vi "PIDF.vi"() -> ()   [LabVIEW 2016]
panel:
  in  "i Zone":dbl format="%.2f"
  in  "Feed Forward":dbl format="%.2f"
  out "output":dbl format="%.2f"
  in  "setpoint":dbl format="%.2f"
  in  "process variable":dbl format="%.2f"
  in  "PIDF gains":cluster{"Kp":dbl, "Ki":dbl, "Kd":dbl, "Kf":dbl}={"Kp"=1.0, "Ki"=0.01, "Kd"=0.0, "Kf"=1.0} {"Kf" format="%.3f"; "Kd" format="%.3f"; "Ki" format="%.3f"; "Kp" format="%.3f"}
  in  "dt (s)":dbl=-1.0 format="%.3f"
  in  "output range":cluster{"output high":dbl, "output low":dbl}={"output high"=1.0, "output low"=-1.0} {"output low" format="%.2f"; "output high" format="%.2f"}
  in  "reinitialize? (F)":bool
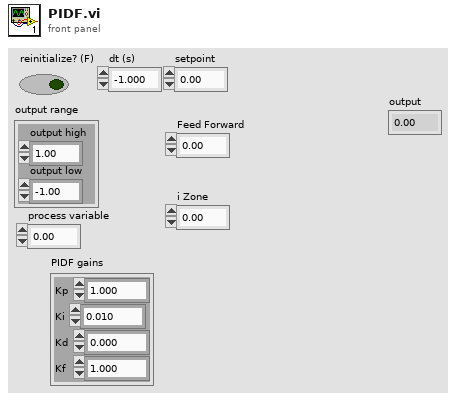
[diagram p1: front panel]
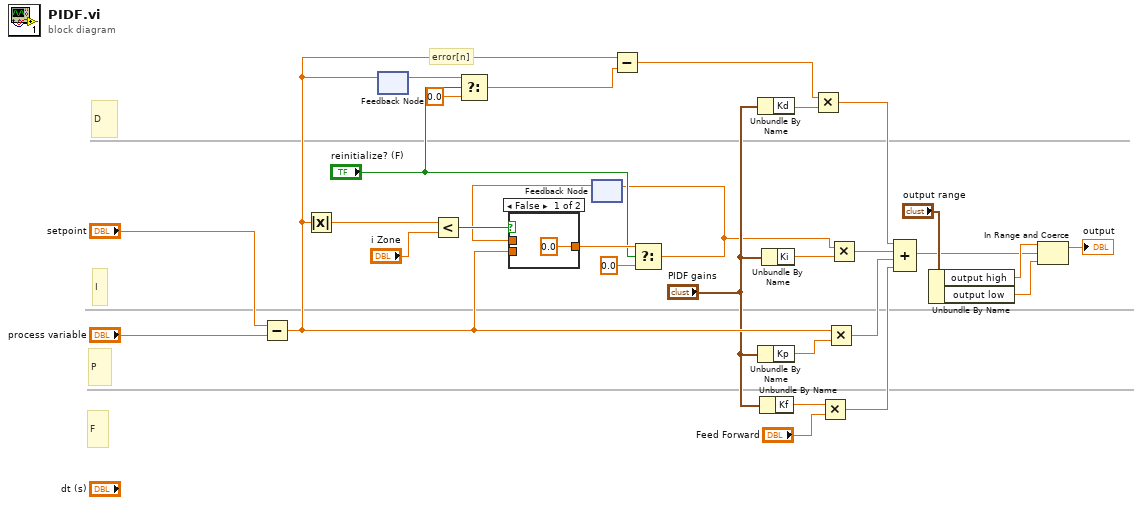
[diagram p0: block diagram]
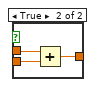
[diagram p2: hidden frame]
diagram:
  # "F"
  # "D"
  # "I"
  # "P"
  # "error[n]"
  n1 = Subtract(x="setpoint", y="process variable") -> (x-y=w20:dbl)
  n2 = Absolute Value(x=w20) -> (abs(x)=w27:dbl)
  n3 = feedback #1() -> (w18:dbl)  [unwired: 1 in]
  n4 = feedback-in #1(w20) -> ()
  n5 = Less?(x=w27, y="i Zone") -> (x < y?=w25:bool)
  n6 = Select(t=w18, s="reinitialize? (F)", f=0.0) -> (s? t:f=w17:dbl)
  n7 = feedback #2() -> (w24:dbl)  [unwired: 1 in]
  n8 = case shown="False" w25 {
    tunnel: w20 -> [_ w34]
    tunnel: [0.0 ("f") w33] -> w23
    tunnel: w24 -> [_ w32]
    frame False {
    }
    frame True {
      n9 = Add(x=w32, y=w34) -> (x+y=w33:dbl)
    }
  }
  n10 = Subtract(x=w20, y=w17) -> (x-y=w5:dbl)
  n11 = Select(t=w23, s="reinitialize? (F)", f=0.0) -> (s? t:f=w2:dbl)
  n12 = feedback-in #2(w2) -> ()
  n13 = Unbundle By Name("PIDF gains") -> ("Kd"=w6:dbl)
  n14 = Unbundle By Name("PIDF gains") -> ("Kp"=w28:dbl)
  n15 = Unbundle By Name("PIDF gains") -> ("Kf"=w9:dbl)
  n16 = Unbundle By Name("PIDF gains") -> ("Ki"=w3:dbl)
  n17 = Multiply(x=w5, y=w6) -> (x*y=w4:dbl)
  n18 = Multiply(x=w9, y="Feed Forward") -> (x*y=w7:dbl)
  n19 = Multiply(x=w20, y=w28) -> (x*y=w16:dbl)
  n20 = Multiply(x=w2, y=w3) -> (x*y=w1:dbl)
  n21 = Compound Arithmetic op=ADD(w4, w1, w16, w7) -> (w11:dbl)
  n22 = Unbundle By Name("output range") -> ("output high"=w13:dbl, "output low"=w12:dbl)
  n23 = In Range and Coerce(upper limit=w13, x=w11, lower limit=w12) -> (coerced(x)=→"output":dbl)  [unwired: 1 out]
